vi "Scripting_RewireSubVISourcesDrains.vi"(8 "error in":errorcluster, 9 "DrainsSources":T2(array[cluster]), 10 "SourceDrains":T1(array[cluster]), 11 "SubVIIn":refnum<vi>) -> (0 "error out":errorcluster)   [LabVIEW 2016]
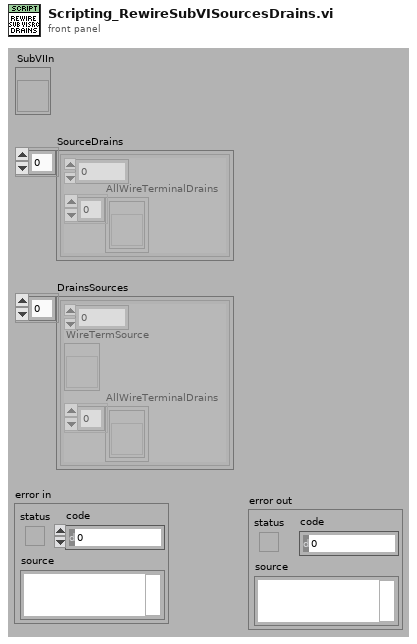
[diagram p1: front panel]
types:
  T1 = cluster{i32, "AllWireTerminalDrains":refnum<vi>[]}[]
  T2 = cluster{i32, "WireTermSource":refnum<vi>, "AllWireTerminalDrains":refnum<vi>[]}[]
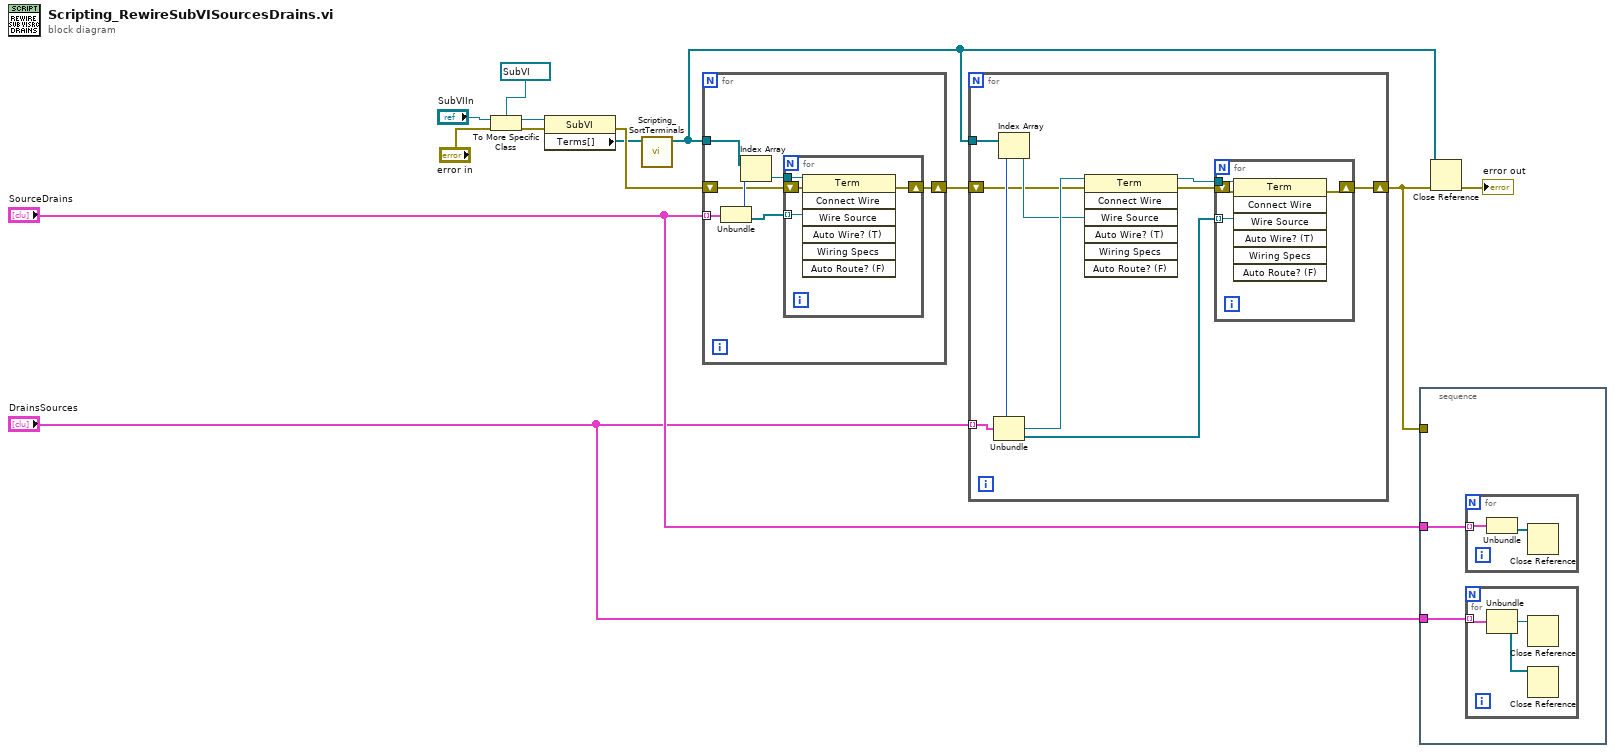
[diagram p0: block diagram]
diagram:
  n1 = To More Specific Class(target class=refnum<vi> refnum ("Block Diagram"), reference="SubVIIn", error in="error in") -> (specific class reference=w2:refnum<vi>, error out=w1:errorcluster)
  n2 = property class="SubVI"(reference=w2, error in=w1) -> (error out=w12:errorcluster, "Terms[]"=w11:refnum<vi>[])  [unwired: 1 out]
  n3 = call <resource>:"Scripting_SortTerminals.vi"("Terminals[]"=w11) -> ("TerminalsOut[]"=w9:refnum<vi>[])  [unwired: 8 in, 2 out]
  n4 = for {
    tunnel: w9 -> [w19]
    tunnel: "SourceDrains" -> [w20] mode=indexing
    shift-right: [w14] -> w13
    shift-left: w12 -> [w15]
    n5 = Unbundle(w20) -> (w18:i32, "AllWireTerminalDrains"=w16:refnum<vi>[])
    n6 = Index Array(array=w19, index=w18) -> (element=w17:refnum<vi>)
    n7 = for {
      tunnel: w17 -> [w24]
      tunnel: w16 -> [w23] mode=indexing
      shift-right: [w21] -> w14
      shift-left: w15 -> [w22]
      n8 = invoke class="Term" method="Connect Wire"(reference=w24, error in=w22, "Wire Source"=w23) -> (error out=w21:errorcluster)  [unwired: 4 in, 6 out]
    }
  }
  n9 = for {
    tunnel: w9 -> [w33]
    tunnel: "DrainsSources" -> [w34] mode=indexing
    shift-right: [w25] -> w8
    shift-left: w13 -> [w27]
    n10 = Unbundle(w34) -> (w32:i32, "WireTermSource"=w31:refnum<vi>, "AllWireTerminalDrains"=w28:refnum<vi>[])
    n11 = Index Array(array=w33, index=w32) -> (element=w30:refnum<vi>)
    n12 = invoke class="Term" method="Connect Wire"(reference=w31, error in=w27, "Wire Source"=w30) -> (reference out=w29:refnum<vi>, error out=w26:errorcluster)  [unwired: 4 in, 5 out]
    n13 = for {
      tunnel: w29 -> [w38]
      tunnel: w28 -> [w37] mode=indexing
      shift-right: [w35] -> w25
      shift-left: w26 -> [w36]
      n14 = invoke class="Term" method="Connect Wire"(reference=w38, error in=w36, "Wire Source"=w37) -> (error out=w35:errorcluster)  [unwired: 4 in, 6 out]
    }
  }
  n15 = stacked-sequence {
    tunnel: w8 -> [_]
    tunnel: "SourceDrains" -> [w40]
    tunnel: "DrainsSources" -> [w39]
    frame #0 {
      n16 = for {
        tunnel: w40 -> [w45] mode=indexing
        n17 = Unbundle(w45) -> ("AllWireTerminalDrains"=w44:refnum<vi>[])  [unwired: 1 out]
        n18 = Close Reference(reference=w44) -> ()  [unwired: 1 in, 1 out]
      }
      n19 = for {
        tunnel: w39 -> [w43] mode=indexing
        n20 = Unbundle(w43) -> ("WireTermSource"=w42:refnum<vi>, "AllWireTerminalDrains"=w41:refnum<vi>[])  [unwired: 1 out]
        n21 = Close Reference(reference=w42) -> ()  [unwired: 1 in, 1 out]
        n22 = Close Reference(reference=w41) -> ()  [unwired: 1 in, 1 out]
      }
    }
  }
  n23 = Close Reference(reference=w9, error in (no error)=w8) -> (error out=→"error out":errorcluster)
